vi "Find and Replace Items.vi"(8 "error in (no error)":errorcluster, 10 "Replace Info":T1={"Filter Column"=enum."Description", "Filter Type"=enum."Contains", "Filter Value"="", "Case Sensitive?"=FALSE, "Replace Column"=enum."Description", "Replace Value"=""}, 11 "New Item Data":refnum<class "Item.lvclass">[](array[class])) -> (0 "error out":errorcluster, 1 "Number of Replacements":i32, 3 "New Item Data out":refnum<class "Item.lvclass">[](array[class]))   [LabVIEW 2020, in "VI Properties Editor.lvlib"]
doc: "Finds and replaces properties of items in <B>New Item Data</B> based on <B>Replace Info</B>."
uses:
  VI Properties Editor.lvlib
  CTLs/Replace Info.ctl
  CTLs/Filter Column.ctl
  CTLs/Filter Type.ctl
  CTLs/Replace Column.ctl
  Classes/Item/Item.lvclass
  Classes/VI/VI.lvclass
  C:/Users/acasalen/Documents/LabVIEW Data/Projects/VI-Properties-Editor/source/Classes/Item/Item.lvclass
  Classes/Control/Control.lvclass
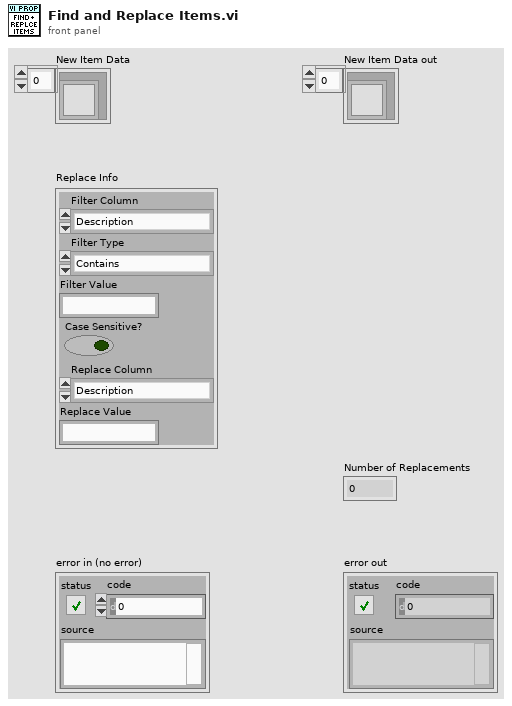
[diagram p1: front panel]
types:
  T1 = typedef "VI Properties Editor.lvlib/Replace Info.ctl" = cluster{"Filter Column":T2, "Filter Type":T3, "Filter Value":string, "Case Sensitive?":bool, "Replace Column":T4, "Replace Value":string}
  T2 = typedef "VI Properties Editor.lvlib/Filter Column.ctl" = enum16{"Name", "Path", "Type", "Window Title", "Description", "Help Path", "Help Tag", "Custom Title?", "Reentrancy", "Inlined?", "Help URL", "Help Type", "Allow Debugging?", "Auto Error Handling?", "Run When Opened?", "Suspend When Called?", "Priority", "Preferred Exec Sytem", "Control Label", "Control Caption", "Control Description", "Control Tip Strip"}
  T3 = typedef "VI Properties Editor.lvlib/Filter Type.ctl" = enum16{"Contains", "Equals", "Starts with", "Ends with", "Is empty", "Does not contain", "Does not equal", "Is not empty"}
  T4 = typedef "VI Properties Editor.lvlib/Replace Column.ctl" = enum16{"Window Title", "Description", "Help Path", "Help Tag", "Custom Title?", "Help URL", "Help Type", "Control Label", "Control Caption", "Control Description", "Control Tip Strip"}
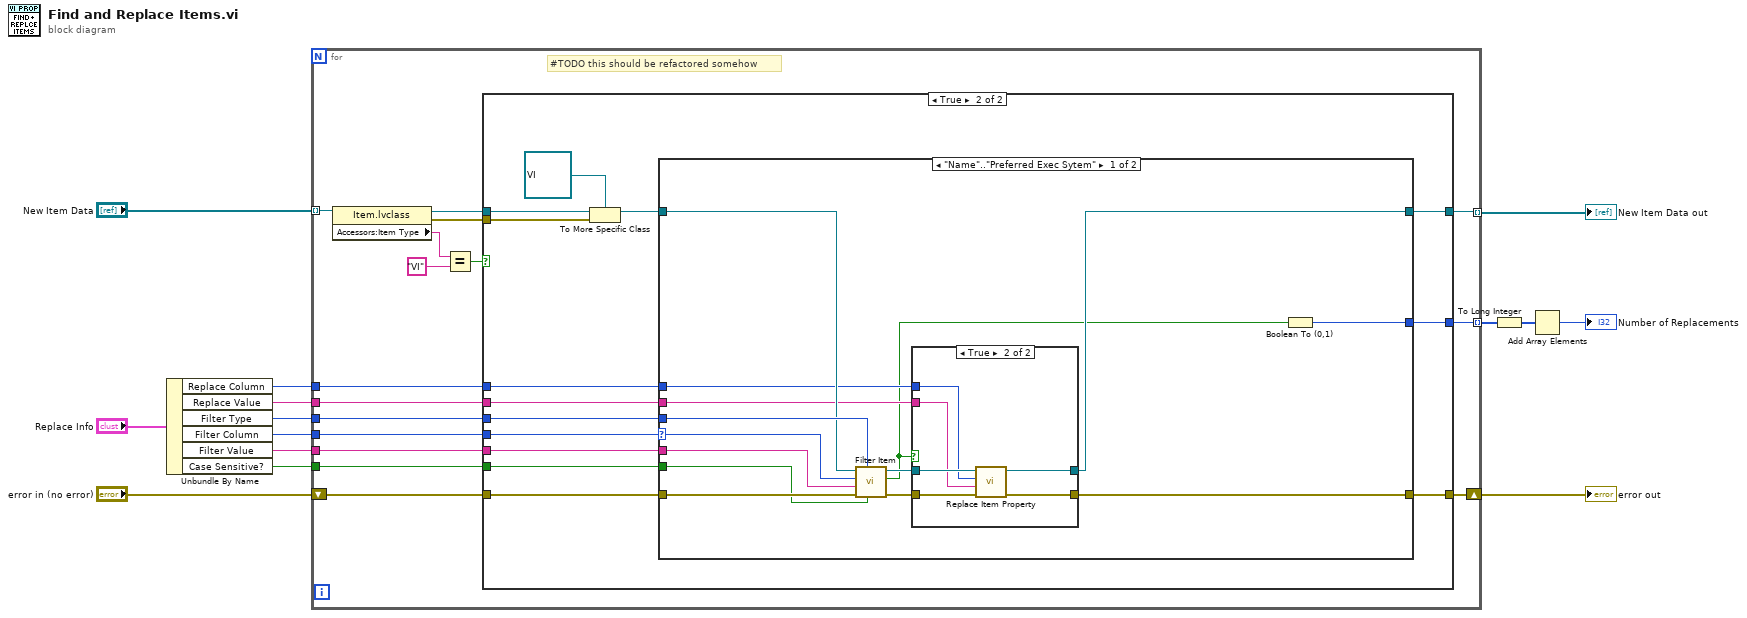
[diagram p0: block diagram]
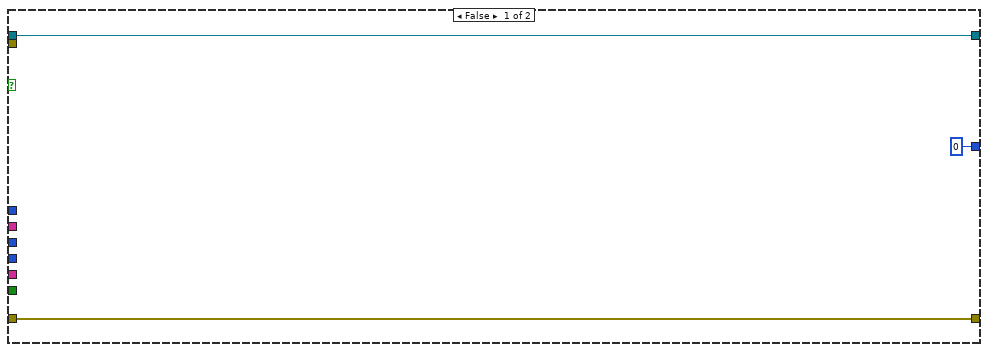
[diagram p2: hidden frame]
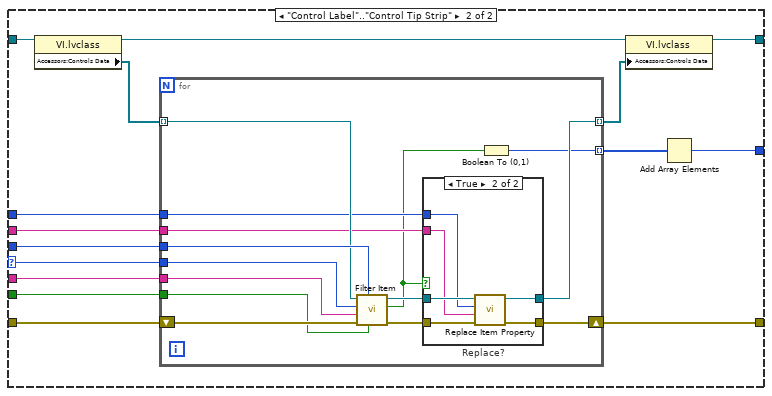
[diagram p4: hidden frame]
diagram:
  n1 = Unbundle By Name("Replace Info") -> ("Replace Column"=w6:T4, "Replace Value"=w7:string, "Filter Type"=w10:T3, "Filter Column"=w9:T2, "Filter Value"=w8:string, "Case Sensitive?"=w1:bool)
  n2 = for {
    tunnel: "New Item Data" -> [w22] mode=indexing
    tunnel: w9 -> [w29]
    tunnel: w10 -> [w27]
    tunnel: w8 -> [w28]
    shift-right: [w18] -> w13
    shift-left: "error in (no error)" -> [w30]
    tunnel: w7 -> [w20]
    tunnel: w6 -> [w19]
    tunnel: [w17] -> w5 mode=indexing
    tunnel: [w16] -> w4 mode=indexing
    tunnel: w1 -> [w15]
    # "#TODO this should be refactored somehow"
    n3 = property class="Item.lvclass"(reference=w22) -> (reference out=w23:refnum<class "Item.lvclass">, error out=w24:errorcluster, "Accessors:Item Type"=w26:string)  [unwired: 1 in]
    n4 = Equal?(x=w26, y="VI") -> (x = y?=w21:bool)
    n5 = case shown="True" w21 {
      tunnel: w30 -> [w33 w47]
      tunnel: w29 -> [_ w46]
      tunnel: w28 -> [_ w45]
      tunnel: w27 -> [_ w44]
      tunnel: w24 -> [_ w43]
      tunnel: w23 -> [w32 w42]
      tunnel: w20 -> [_ w39]
      tunnel: w19 -> [_ w38]
      tunnel: [w33 w37] -> w18
      tunnel: [w32 w36] -> w17
      tunnel: [i16 0 w35] -> w16
      tunnel: w15 -> [_ w34]
      frame False {
      }
      frame True {
        n6 = To More Specific Class(target class=refnum<class "VI.lvclass"> refnum ("VI Properties Editor.lvlib:VI.lvclass"), reference=w42, error in=w43) -> (specific class reference=w40:refnum<class "VI.lvclass">)  [unwired: 1 out]
        n7 = case shown="\"Name\"..\"Preferred Exec Sytem\"" w46 {
          selector: w46 -> [w60 w83]
          tunnel: w47 -> [w61 w84]
          tunnel: w45 -> [w59 w82]
          tunnel: w44 -> [w58 w81]
          tunnel: w40 -> [w57 w80]
          tunnel: [w52 w76] -> w36
          tunnel: w39 -> [w53 w75]
          tunnel: w38 -> [w54 w74]
          tunnel: [w51 w73] -> w37
          tunnel: [w49 w71] -> w35
          tunnel: w34 -> [w48 w70]
          frame "Name".."Preferred Exec Sytem" {
            n8 = call-dynamic "Filter Item.vi"("Case Sensitive?"=w48, "Filter Type"=w58, "error in (no error)"=w61, "Filter Value"=w59, "Filter Column"=w60, "VI in"=w57) -> ("error out"=w56:errorcluster, "Include?"=w50:bool, "VI out"=w55:refnum<class "VI.lvclass">)  [unwired: 3 in]
            n9 = case shown="True" w50 {
              tunnel: w56 -> [w62 w69]
              tunnel: w55 -> [w63 w68]
              tunnel: w54 -> [_ w67]
              tunnel: w53 -> [_ w66]
              tunnel: [w62 w65] -> w51
              tunnel: [w63 w64] -> w52
              frame False {
              }
              frame True {
                n10 = call-dynamic "Replace Item Property.vi"("error in (no error)"=w69, "Replace Value"=w66, "Replace Column"=w67, "VI in"=w68) -> ("error out"=w65:errorcluster, "VI out"=w64:refnum<class "VI.lvclass">)  [unwired: 6 in]
              }
            }
            n11 = Boolean To (0,1)(Boolean=w50) -> (0, 1=w49:i16)
          }
          frame "Control Label".."Control Tip Strip" {
            n12 = property class="VI.lvclass"(reference=w80) -> (reference out=w78:refnum<class "VI.lvclass">, "Accessors:Controls Data"=w79:refnum<class "Control.lvclass">[])  [unwired: 1 in, 1 out]
            n13 = for {
              tunnel: w83 -> [w97]
              tunnel: w82 -> [w96]
              tunnel: w81 -> [w95]
              tunnel: w79 -> [w94] mode=indexing
              shift-right: [w90] -> w73
              shift-left: w84 -> [w98]
              tunnel: [w91] -> w77 mode=indexing
              tunnel: w75 -> [w89]
              tunnel: w74 -> [w88]
              tunnel: [w86] -> w72 mode=indexing
              tunnel: w70 -> [w85]
              n14 = call-dynamic "Filter Item.vi"("Case Sensitive?"=w85, "Filter Type"=w95, "error in (no error)"=w98, "Filter Value"=w96, "Filter Column"=w97, "Control in"=w94) -> ("error out"=w93:errorcluster, "Include?"=w87:bool, "Control out"=w92:refnum<class "Control.lvclass">)  [unwired: 3 in]
              n15 = case "Replace?" shown="True" w87 {
                tunnel: w93 -> [w99 w106]
                tunnel: w92 -> [w100 w105]
                tunnel: w89 -> [_ w104]
                tunnel: w88 -> [_ w103]
                tunnel: [w100 w102] -> w91
                tunnel: [w99 w101] -> w90
                frame False {
                }
                frame True {
                  n16 = call-dynamic "Replace Item Property.vi"("error in (no error)"=w106, "Replace Value"=w104, "Replace Column"=w103, "Control in"=w105) -> ("error out"=w101:errorcluster, "Control out"=w102:refnum<class "Control.lvclass">)  [unwired: 6 in]
                }
              }
              n17 = Boolean To (0,1)(Boolean=w87) -> (0, 1=w86:i16)
            }
            n18 = property class="VI.lvclass"(reference=w78, "Accessors:Controls Data"=w77) -> (reference out=w76:refnum<class "VI.lvclass">)  [unwired: 1 in, 1 out]
            n19 = Add Array Elements(numeric array=w72) -> (sum=w71:i16)
          }
        }
      }
    }
  }
  "New Item Data out" <- w5
  "error out" <- w13
  n20 = To Long Integer(number=w4) -> (32bit integer=w3:i32[])
  n21 = Add Array Elements(numeric array=w3) -> (sum=→"Number of Replacements":i32)
